vi "Actor Core.vi"(8 "error in":errorcluster, 11 "TDMS DAQ in":refnum<class "TDMS DAQ.lvclass">) -> (0 "error out":errorcluster, 3 "Actor out":refnum<class "Actor.lvclass">)   [LabVIEW 2020, in "TDMS DAQ.lvlib" / "TDMS DAQ.lvclass"]
doc: "<p>(<strong>Filename</strong>: <span class=\"dnl\">Actor Framework.lvlib:Actor.lvclass:Actor Core.vi</span>)</p>\n<p>Receives messages to the actor, reacts to them, and initiates any error handling that may shut the actor down.</p>\n<p>Descendant classes may override this VI to append parallel tasks for the actor to complete while it handles messages. Overrides use the <a href=\"nihelplauncher://docs/csh?context=lvcore_glang_udclass\">Call Parent Class Method</a> node.</p>"
uses:
  TDMS DAQ.lvclass
  <vilib>/ActorFramework/Actor/Actor.lvclass
  Helper Loop Message.ctl
  Helper Loop Type.ctl
  TDMS DAQ.lvclass/TDMS DAQ.ctl
  DAQ Interface/DAQ Interface/DAQ Interface.lvclass
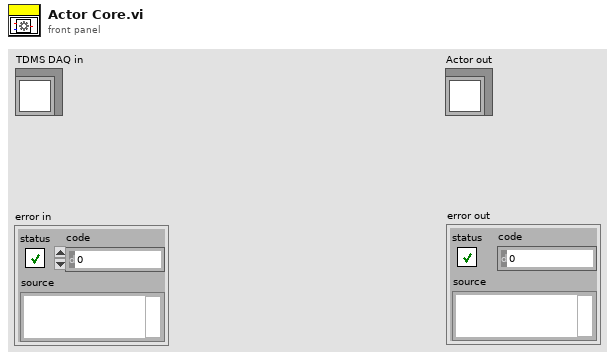
[diagram p1: front panel]
types:
  T1 = typedef "TDMS DAQ.lvlib/TDMS DAQ.lvclass/Helper Loop Message.ctl" = cluster{"Type":T2, "Payload":variant}
  T2 = typedef "TDMS DAQ.lvlib/TDMS DAQ.lvclass/Helper Loop Type.ctl" = enum16{"Configure", "Start", "Do", "Stop", "Clean", "Close"}
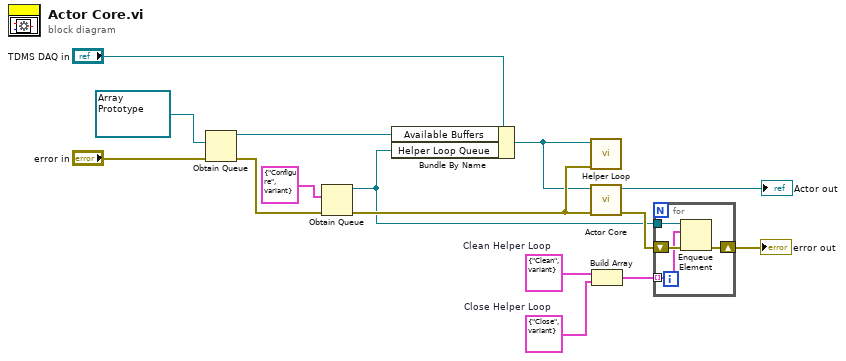
[diagram p0: block diagram]
diagram:
  w5 = T1 {"Type"=enum."Close", "Payload"=variant}  # Close Helper Loop
  w7 = T1 {"Type"=enum."Clean", "Payload"=variant}  # Clean Helper Loop
  n1 = Obtain Queue(element data type=refnum<data-value> refnum ("DMA Memory"), error in (no error)="error in") -> (queue out=w4:refnum<queue>, error out=w3:errorcluster)  [unwired: 3 in, 1 out]
  n2 = Obtain Queue(element data type=T1 {"Type"=enum."Configure", "Payload"=variant} ("Message"), error in (no error)=w3) -> (queue out=w9:refnum<queue>, error out=w12:errorcluster)  [unwired: 3 in, 1 out]
  n3 = Bundle By Name(cluster="TDMS DAQ in", "Available Buffers"=w4, "Helper Loop Queue"=w9) -> (w11:refnum<class "TDMS DAQ.lvclass">)
  n4 = call "Helper Loop.vi"("error in (no error)"=w12, "TDMS DAQ in"=w11) -> ()  [unwired: 10 in]
  n5 = call-parent "Actor Core.vi"("error in"=w12, "Actor in"=w11) -> ("error out"=w10:errorcluster, "Actor out"=→"Actor out":refnum<class "Actor.lvclass">)  [unwired: 8 in]
  n6 = Build Array(w7, w5) -> (w6:T1[])
  n7 = for {
    tunnel: w9 -> [w18]
    tunnel: w6 -> [w16] mode=indexing
    shift-right: [w17] -> w8
    shift-left: w10 -> [w19]
    n8 = Enqueue Element(queue=w18, element=w16, error in (no error)=w19) -> (error out=w17:errorcluster)  [unwired: 1 in, 2 out]
  }
  "error out" <- w8
